vi "run_event.vi"() -> ()   [LabVIEW 2011]
uses:
  Dependencies/global.vi
panel:
  out "Sent data":string
  out "Current Time":string
  out "Events":i32[][](array[numeric])
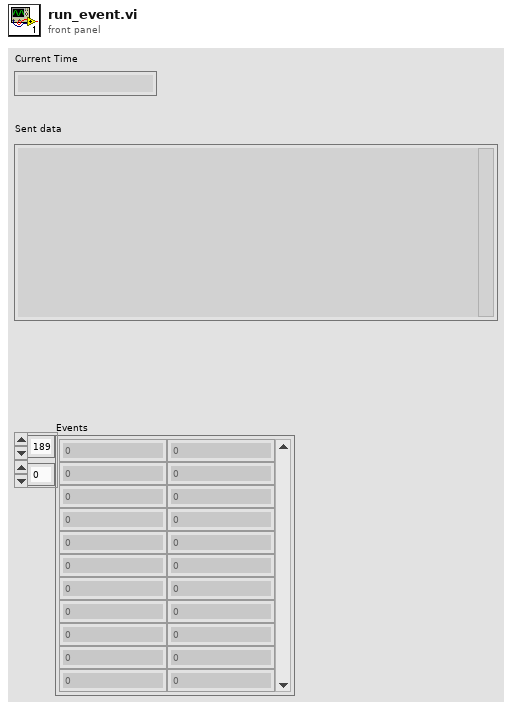
[diagram p1: front panel]
types:
  T1 = cluster{string, string, string, string, string, string, string, string}
  T2 = cluster{string, string, string, string, string, "date/time string":string, string, string}
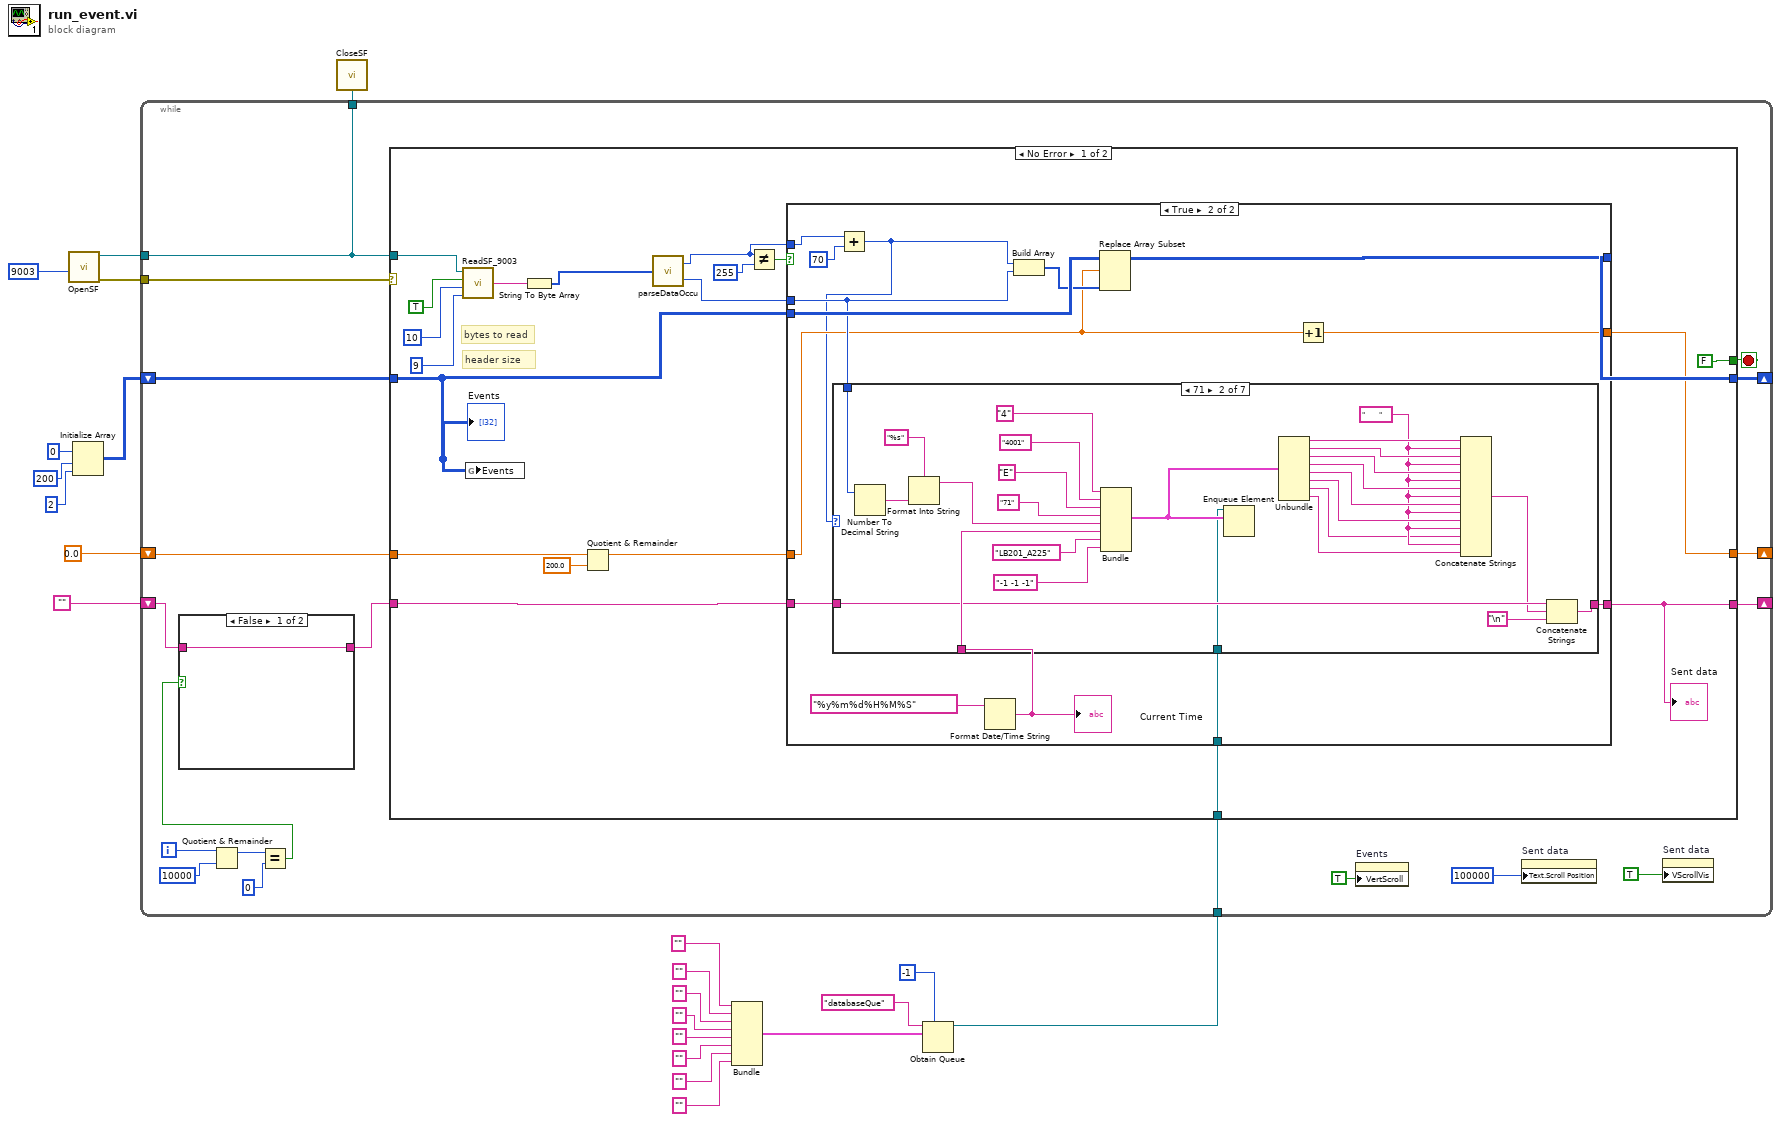
[diagram p0: block diagram]
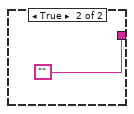
[diagram p2: hidden frame]
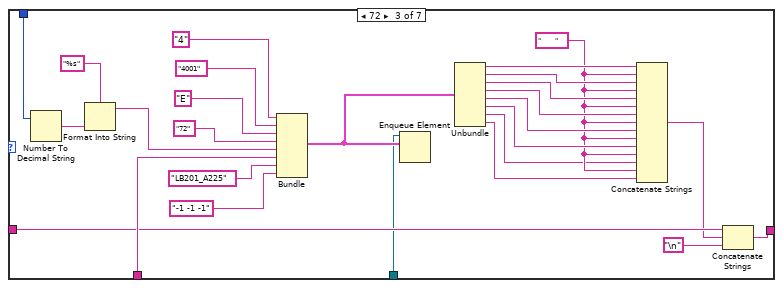
[diagram p5: hidden frame]
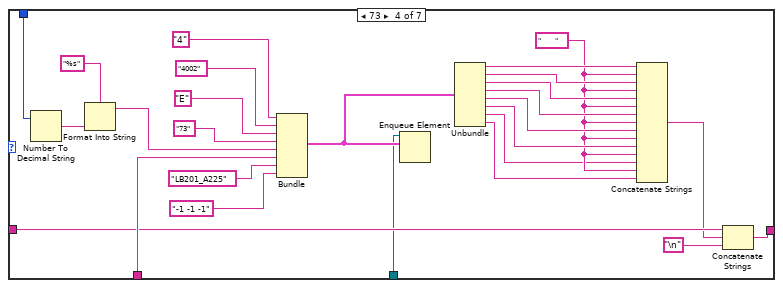
[diagram p6: hidden frame]
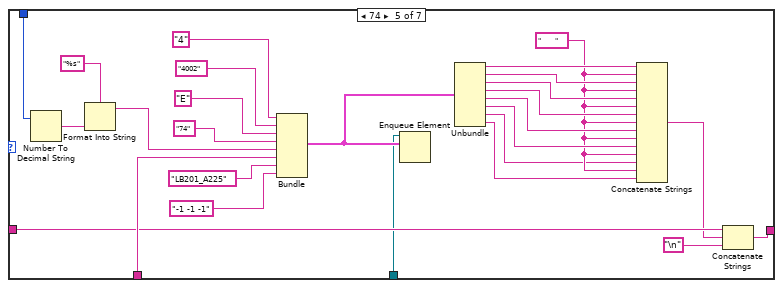
[diagram p7: hidden frame]
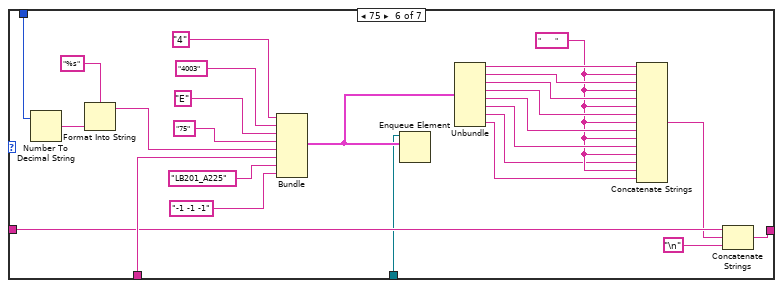
[diagram p8: hidden frame]
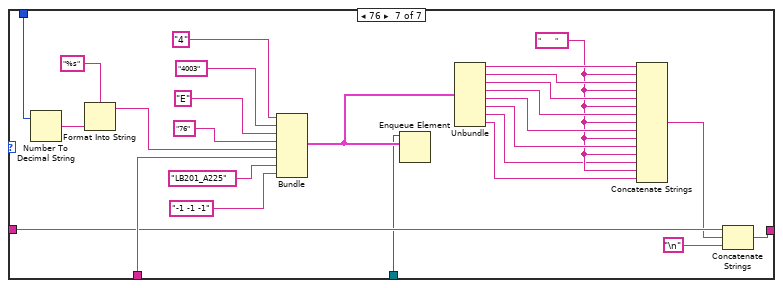
[diagram p9: hidden frame]
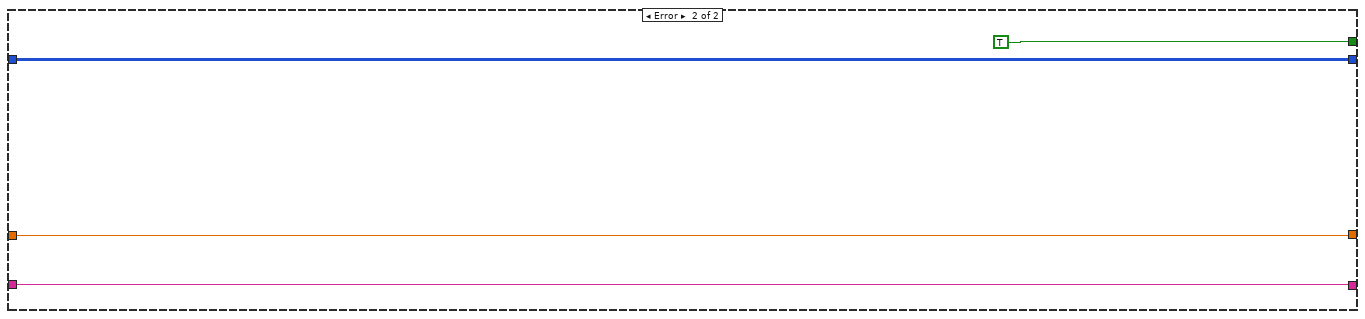
[diagram p10: hidden frame]
diagram:
  n1 = call "OpenSF.vi"("port number"=u16 9003) -> ("error out"=w9:errorcluster, "connection ID"=w10:refnum<k5>)  [unwired: 1 out]
  n2 = Initialize Array(0 ("bytes to read"), 200 ("dimension size"), 2 ("dimension size")) -> (w4:i32[][])
  n3 = Bundle("", "", "", "", "", "", "", "") -> (w19:T1)  [unwired: 1 in]
  n4 = Obtain Queue(max queue size (-1, unlimited)=-1, name (unnamed)="databaseQue", element data type=w19) -> (queue out=w6:refnum<queue>)  [unwired: 2 in, 2 out]
  n5 = while {
    tunnel: w10 -> [w41]
    tunnel: w9 -> [w39]
    tunnel: [w41] -> w8
    shift-right: [w37] -> _
    shift-left: w4 -> [w38]
    shift-right: [w36] -> _
    shift-left: "" -> [w23]
    tunnel: w6 -> [w35]
    shift-right: [w31] -> _
    shift-left: 0.0 -> [w30]
    i -> [w29]
    stop <- w40 stop-if-true
    n6 = Quotient & Remainder(x=w29, y=10000) -> (x-y*floor(x/y)=w27:i32)  [unwired: 1 out]
    n7 = Equal?(x=w27, y=0) -> (x = y?=w25:bool)
    n8 = case shown="False" w25 {
      tunnel: [w42 ""] -> w24
      tunnel: w23 -> [w42 _]
      frame False {
      }
      frame True {
      }
    }
    n9 = case shown="No Error" w39 {
      tunnel: w41 -> [w59 _]
      tunnel: [FALSE TRUE] -> w40
      tunnel: w38 -> [w48 w240]
      tunnel: [w54 w240] -> w37
      tunnel: w24 -> [w57 w239]
      tunnel: [w55 w239] -> w36
      tunnel: w35 -> [w56 _]
      tunnel: [w47 w238] -> w31
      tunnel: w30 -> [w45 w238]
      frame No Error {
        # "header size"
        # "bytes to read"
        n10 = call "ReadSF_9003.vi"("connection ID in"=w59, "enabled"=TRUE, "bytes to read"=10, "header size"=9) -> ("string"=w60:string)  [unwired: 2 in, 2 out]
        n11 = global write "global.vi" "Events"(w48) -> ()
        n12 = String To Byte Array(string=w60) -> (unsigned byte array=w49:u8[])
        n13 = Quotient & Remainder(x=w45, y=200.0) -> (x-y*floor(x/y)=w46:dbl)  [unwired: 1 out]
        n14 = call "parseDataOccu.vi"("array"=w49) -> ("Event (1 bytes)"=w52:u16, "TS (4  bytes)"=w51:u32)
        n15 = Not Equal?(x=w52, y=u16 255) -> (x != y?=w53:bool)
        n16 = case shown="True" w53 {
          tunnel: w52 -> [_ w69]
          tunnel: w51 -> [_ w77]
          tunnel: w48 -> [w66 w80]
          tunnel: [w66 w79] -> w54
          tunnel: w57 -> [w65 w76]
          tunnel: [w65 w75] -> w55
          tunnel: w56 -> [_ w72]
          tunnel: w46 -> [w64 w70]
          tunnel: [w64 w71] -> w47
          frame False {
          }
          frame True {
            n17 = Add(x=w69, y=u16 70) -> (x+y=w67:u16)
            n18 = Format Date/Time String(time format string (%c)="%y%m%d%H%M%S") -> (date/time string=w73:string)  [unwired: 2 in]
            "Current Time" <- w73
            n19 = case shown="71" w67 {
              tunnel: w73 -> [_ w107 w133 w159 w185 w211 w237]
              tunnel: w76 -> [w81 w106 w132 w158 w184 w210 w236]
              tunnel: [w81 w105 w131 w157 w183 w209 w235] -> w75
              tunnel: w77 -> [_ w83 w108 w135 w160 w187 w212]
              tunnel: w72 -> [_ w82 w109 w134 w161 w186 w213]
              frame 0, Default {
              }
              frame 71 {
                w87 = "       "
                n20 = Number To Decimal String(number=w83) -> (decimal integer string=w84:string)  [unwired: 1 in]
                n21 = Format Into String(format string="%s", w84) -> (resulting string=w91:string)  [unwired: 2 in, 1 out]
                n22 = Bundle("4", "4001", "E", "71", w91, "date/time string"=w107, "LB201_A225", "-1 -1 -1") -> (w97:T2)  [unwired: 1 in]
                n23 = Enqueue Element(queue=w82, element=w97) -> ()  [unwired: 2 in, 3 out]
                n24 = Unbundle(w97) -> (w103:string, w102:string, w101:string, w100:string, w99:string, "date/time string"=w98:string, w86:string, w85:string)
                n25 = Concatenate Strings(w103, w87, w102, w87, w101, w87, w100, w87, w99, w87, w98, w87, w86, w87, w85) -> (w95:string)
                n26 = Concatenate Strings(w106, w95, "\n") -> (w105:string)
              }
              frame 72 {
                w113 = "       "
                n27 = Number To Decimal String(number=w108) -> (decimal integer string=w110:string)  [unwired: 1 in]
                n28 = Format Into String(format string="%s", w110) -> (resulting string=w117:string)  [unwired: 2 in, 1 out]
                n29 = Bundle("4", "4001", "E", "72", w117, "date/time string"=w133, "LB201_A225", "-1 -1 -1") -> (w123:T2)  [unwired: 1 in]
                n30 = Enqueue Element(queue=w109, element=w123) -> ()  [unwired: 2 in, 3 out]
                n31 = Unbundle(w123) -> (w129:string, w128:string, w127:string, w126:string, w125:string, "date/time string"=w124:string, w112:string, w111:string)
                n32 = Concatenate Strings(w129, w113, w128, w113, w127, w113, w126, w113, w125, w113, w124, w113, w112, w113, w111) -> (w121:string)
                n33 = Concatenate Strings(w132, w121, "\n") -> (w131:string)
              }
              frame 73 {
                w139 = "       "
                n34 = Number To Decimal String(number=w135) -> (decimal integer string=w136:string)  [unwired: 1 in]
                n35 = Format Into String(format string="%s", w136) -> (resulting string=w143:string)  [unwired: 2 in, 1 out]
                n36 = Bundle("4", "4002", "E", "73", w143, "date/time string"=w159, "LB201_A225", "-1 -1 -1") -> (w149:T2)  [unwired: 1 in]
                n37 = Enqueue Element(queue=w134, element=w149) -> ()  [unwired: 2 in, 3 out]
                n38 = Unbundle(w149) -> (w155:string, w154:string, w153:string, w152:string, w151:string, "date/time string"=w150:string, w138:string, w137:string)
                n39 = Concatenate Strings(w155, w139, w154, w139, w153, w139, w152, w139, w151, w139, w150, w139, w138, w139, w137) -> (w147:string)
                n40 = Concatenate Strings(w158, w147, "\n") -> (w157:string)
              }
              frame 74 {
                w165 = "       "
                n41 = Number To Decimal String(number=w160) -> (decimal integer string=w162:string)  [unwired: 1 in]
                n42 = Format Into String(format string="%s", w162) -> (resulting string=w169:string)  [unwired: 2 in, 1 out]
                n43 = Bundle("4", "4002", "E", "74", w169, "date/time string"=w185, "LB201_A225", "-1 -1 -1") -> (w175:T2)  [unwired: 1 in]
                n44 = Enqueue Element(queue=w161, element=w175) -> ()  [unwired: 2 in, 3 out]
                n45 = Unbundle(w175) -> (w181:string, w180:string, w179:string, w178:string, w177:string, "date/time string"=w176:string, w164:string, w163:string)
                n46 = Concatenate Strings(w181, w165, w180, w165, w179, w165, w178, w165, w177, w165, w176, w165, w164, w165, w163) -> (w173:string)
                n47 = Concatenate Strings(w184, w173, "\n") -> (w183:string)
              }
              frame 75 {
                w191 = "       "
                n48 = Number To Decimal String(number=w187) -> (decimal integer string=w188:string)  [unwired: 1 in]
                n49 = Format Into String(format string="%s", w188) -> (resulting string=w195:string)  [unwired: 2 in, 1 out]
                n50 = Bundle("4", "4003", "E", "75", w195, "date/time string"=w211, "LB201_A225", "-1 -1 -1") -> (w201:T2)  [unwired: 1 in]
                n51 = Enqueue Element(queue=w186, element=w201) -> ()  [unwired: 2 in, 3 out]
                n52 = Unbundle(w201) -> (w207:string, w206:string, w205:string, w204:string, w203:string, "date/time string"=w202:string, w190:string, w189:string)
                n53 = Concatenate Strings(w207, w191, w206, w191, w205, w191, w204, w191, w203, w191, w202, w191, w190, w191, w189) -> (w199:string)
                n54 = Concatenate Strings(w210, w199, "\n") -> (w209:string)
              }
              frame 76 {
                w217 = "       "
                n55 = Number To Decimal String(number=w212) -> (decimal integer string=w214:string)  [unwired: 1 in]
                n56 = Format Into String(format string="%s", w214) -> (resulting string=w221:string)  [unwired: 2 in, 1 out]
                n57 = Bundle("4", "4003", "E", "76", w221, "date/time string"=w237, "LB201_A225", "-1 -1 -1") -> (w227:T2)  [unwired: 1 in]
                n58 = Enqueue Element(queue=w213, element=w227) -> ()  [unwired: 2 in, 3 out]
                n59 = Unbundle(w227) -> (w233:string, w232:string, w231:string, w230:string, w229:string, "date/time string"=w228:string, w216:string, w215:string)
                n60 = Concatenate Strings(w233, w217, w232, w217, w231, w217, w230, w217, w229, w217, w228, w217, w216, w217, w215) -> (w225:string)
                n61 = Concatenate Strings(w236, w225, "\n") -> (w235:string)
              }
            }
            n62 = Build Array(w67, w77) -> (w78:u32[])
            n63 = Replace Array Subset(array=w80, new element=w78, index (row)=w70) -> (w79:i32[][])  [unwired: 1 in]
            n64 = Increment(x=w70) -> (x+1=w71:dbl)
          }
        }
        "Sent data" <- w55
        "Events" <- w48
      }
      frame Error {
      }
    }
    n65 = property on="Events" class="Arr (strict)"("VertScroll"=TRUE ("Vertical Scrollbar Visible")) -> ()  [unwired: 2 in, 2 out]
    n66 = property on="Sent data" class="Str"("Text.Scroll Position"=u32 100000) -> ()  [unwired: 2 in, 2 out]
    n67 = property on="Sent data" class="Str"("VScrollVis"=TRUE ("Vertical Scrollbar Visible")) -> ()  [unwired: 2 in, 2 out]
  }
  n68 = call "CloseSF.vi"("connection ID"=w8) -> ()  [unwired: 2 in]
